vi "Build Group Status Map.vi"(8 "error in (no error)":errorcluster, 10 "Descendants":refnum<class "Config Element.lvclass">[](array[class])) -> (0 "error out":errorcluster, 2 "Map":T1(c390))   [LabVIEW 2020, in "VolatusGUIElements.lvlib" / "GroupLoggingControl.lvclass"]
uses:
  GroupLoggingControl.lvclass
  GroupLoggingControl.lvclass/GroupLoggingControl.ctl
  lv-cdm/CDM-Config/Config Element/Config Element.lvclass
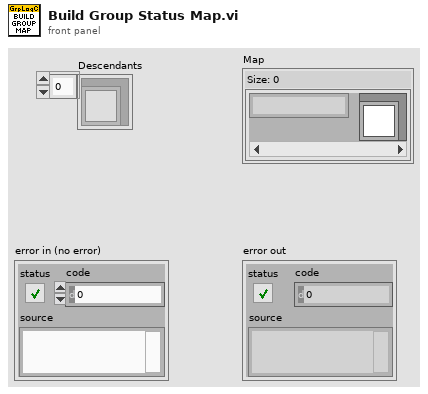
[diagram p1: front panel]
types:
  T1 = map{string, refnum<class "Config Element.lvclass">}
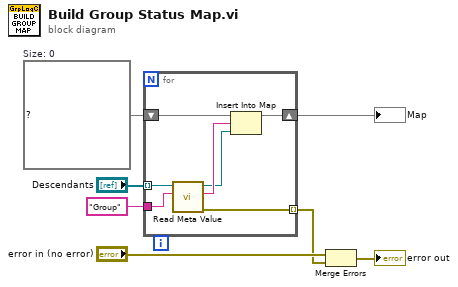
[diagram p0: block diagram]
diagram:
  w5 = T1 {}  # Size: 0
  n1 = for {
    tunnel: "Descendants" -> [w14] mode=indexing
    tunnel: "Group" ("Meta Name") -> [w13]
    shift-right: [w9] -> w4
    shift-left: w5 -> [w12]
    tunnel: [w8] -> w1 mode=indexing
    n2 = call "Read Meta Value.vi"("Meta Name"=w13, "Config Element in"=w14) -> ("error out"=w8:errorcluster, "Meta Value"=w11:string, "Config Element out"=w10:refnum<class "Config Element.lvclass">)  [unwired: 7 in]
    n3 = Insert Into Map(map in=w12, key=w11, value=w10) -> (map out=w9:T1)  [unwired: 2 out]
  }
  "Map" <- w4
  n4 = Merge Errors("error in (no error)", w1) -> (→"error out":errorcluster)
